vi "Create Data File.vi"(8 "error in (no error)":errorcluster, 9 "File Type":string, 11 "Data File I/O Information":T1={"Name of Configuration"="", "Path"=path "C:/Users/Achilles/Data/12-20-00", "File Name"="Whole Gel Image", "Files To Acquire"=1, "Current File Number"=21, "Time Limit"=1.0, "Save Data"=FALSE, "Additional Comments"=""}) -> (0 "error out":errorcluster, 1 "new file path":path, 2 "refnum":refnum<file>, 3 "Data File I/O Information":T1={"Name of Configuration"="", "Path"=path "C:/Users/Achilles/Data/12-20-00", "File Name"="Whole Gel Image", "Files To Acquire"=1, "Current File Number"=21, "Time Limit"=1.0, "Save Data"=FALSE, "Additional Comments"=""}, 4 "First section offset":i32, 6 "Offset for index pointer":i32)   [LabVIEW 2009]
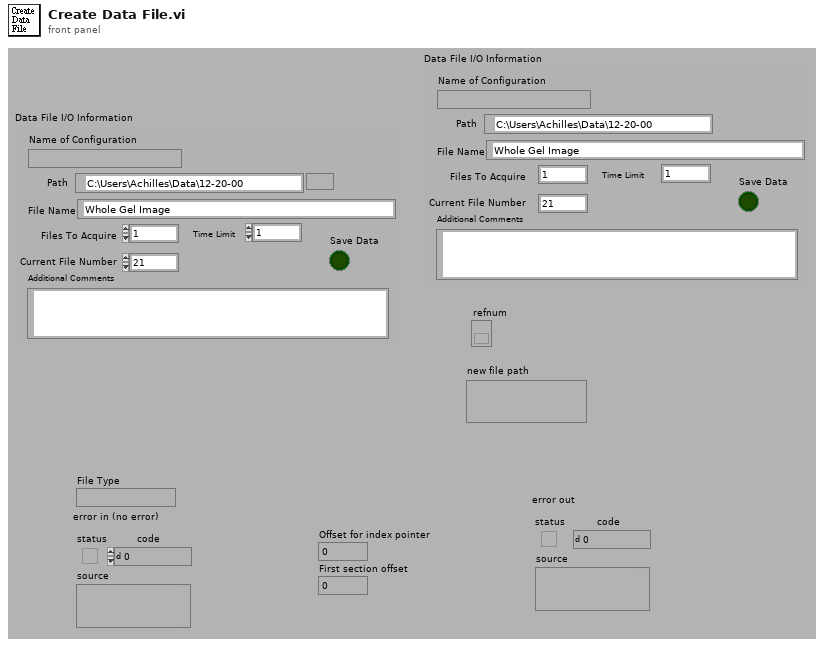
[diagram p1: front panel]
types:
  T1 = cluster{"Name of Configuration":string, "Path":path, "File Name":string, "Files To Acquire":i32, "Current File Number":i32, "Time Limit":dbl, "Save Data":bool, "Additional Comments":string}
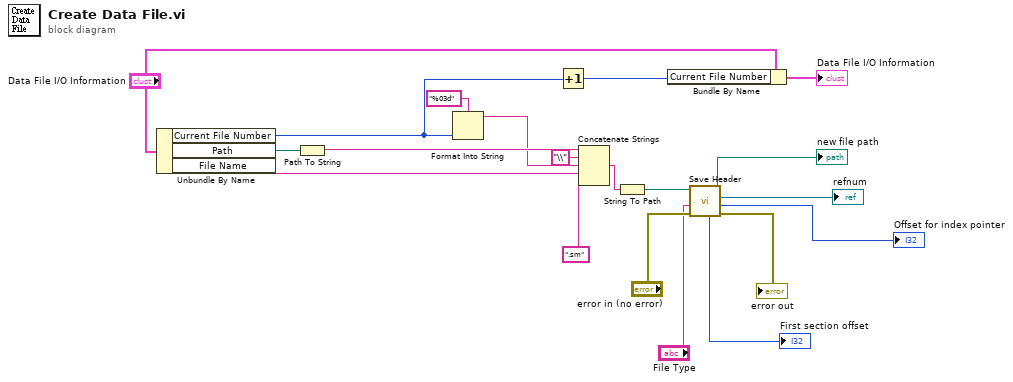
[diagram p0: block diagram]
diagram:
  n1 = Unbundle By Name("Data File I/O Information") -> ("Current File Number"=w18:i32, "Path"=w16:path, "File Name"=w7:string)
  n2 = Path To String(path=w16) -> (string=w10:string)
  n3 = Format Into String(format string="%03d" ("Format String"), w18) -> (resulting string=w8:string)  [unwired: 2 in, 1 out]
  n4 = Increment(x=w18) -> (x+1=w19:i32)
  n5 = Concatenate Strings(w10, "\\" ("Substring"), w8, w7, ".sm" ("Substring")) -> (w15:string)
  n6 = String To Path(string=w15) -> (path=w12:path)
  n7 = Bundle By Name(cluster="Data File I/O Information", "Current File Number"=w19) -> (→"Data File I/O Information":T1)
  n8 = call "Save Header.vi"("error in (no error)"="error in (no error)", "File Type"="File Type", "Configuration Path"=w12) -> ("error out"=→"error out":errorcluster, "Offset for index pointer"=→"Offset for index pointer":i32, "refnum"=→"refnum":refnum<file>, "new file path"=→"new file path":path, "First section offset"=→"First section offset":i32)  [unwired: 4 in]
